vi "Init.vi"(8 "error in (no error)":errorcluster, 11 "Ingredient":T1) -> (0 "error out":errorcluster, 3 "Item Summary out":refnum<class "Item Summary.lvclass">)   [LabVIEW 2020]
uses:
  Item Summary.lvclass
  C:/dev/LabVIEW/lv-oopanel/OOPanel/ArrayPanel/ArrayPanel.lvclass
  C:/dev/LabVIEW/lv-oopanel/OOPanel/Panel/Panel.lvclass
  C:/dev/LabVIEW/Good Company Calc/Item Summary/Item Summary.lvclass
  Item/Item.lvclass
  Item/Ingredient.ctl
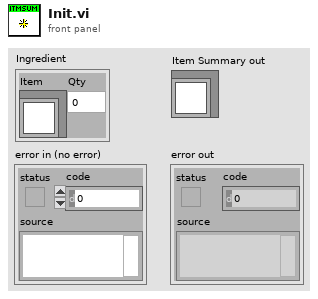
[diagram p1: front panel]
types:
  T1 = typedef "Item.lvclass/Ingredient.ctl" = cluster{"Item":refnum<class "Item.lvclass">, "Qty":dbl}
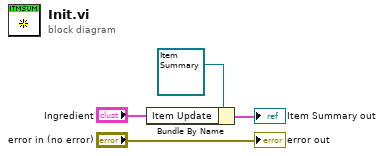
[diagram p0: block diagram]
diagram:
  n1 = Bundle By Name(cluster=refnum<class "Item Summary.lvclass"> refnum ("Item Summary in"), "Item Update"="Ingredient") -> (→"Item Summary out":cluster{})
  "error out" <- "error in (no error)"
